vi "E709_Sample_Application_2a.vi"(11 "error in":errorcluster) -> (15 "error out":errorcluster)   [LabVIEW 2014, in "PiFOC.lvlib"]
doc: "This VI demonstrates how to statically define an E-709 configuration with two E 709 controllers. \nIn this example, the first E-709 is connected through COM port 1 with baudrate 115200 and the second through USB with an unknown serial number (Search? = TRUE). The VI runs \"E709_Configuration_Setup.vi\" for both controllers with these pre-defined settings and reads the position of the axes. The diagram shows how to combine the driver VIs for these tasks.\n\nWarning: This VI has Interface settings for each controller that probably do not match your current configuration. Please modify the \"Interface\", \"RS232 settings\" or \"USB settings\" in the diagram before running the VI."
uses:
  PiFOC.lvlib
panel:
  in  "stop":bool
  out "Position system 2":dbl[](array[numeric]) format="%.6f"
  out "Identification E-709 controller 2":string
  out "Conn. Axis system 2":string[](array[string])
  out "Running":bool caption="Axes are referencing"
  out "Position system 1":dbl[](array[numeric]) format="%.6f"
  out "Conn. Axis system 1":string[](array[string])
  out "Identification E-709 controller 1":string
  # "Simple E-709 sample program"
  # "This VI demonstrates how to statically define an E-709 configuration with two E-709 controllers. In this example, the first E-709 is connected through COM\nport 1 with baudrate 57600 and the second through USB. The VI runs E709_Configuration_Setup.vi for both controllers with these pre-defined settings \nand reads the position of the axes. The diagram shows how to combine the driver VIs for these tasks. \n\nWarning: This VI has Interface settings for each controller that probably do not match your current configuration. Please modify the \n                 \"Interface\", \"RS232 settings\" or USB settings\" in the diagram before running the VI."
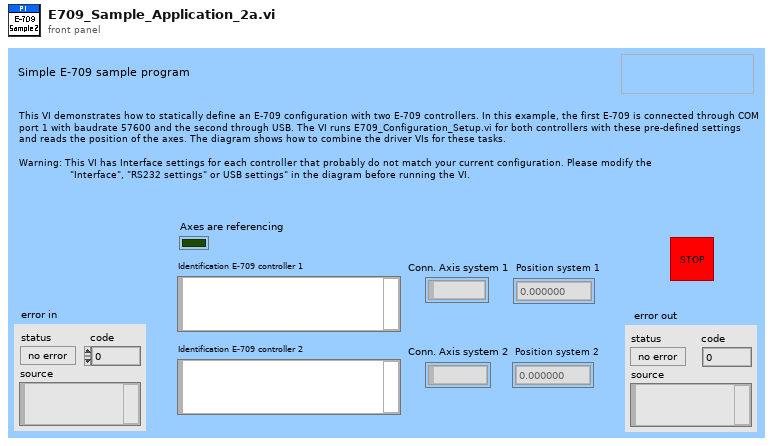
[diagram p1: front panel]
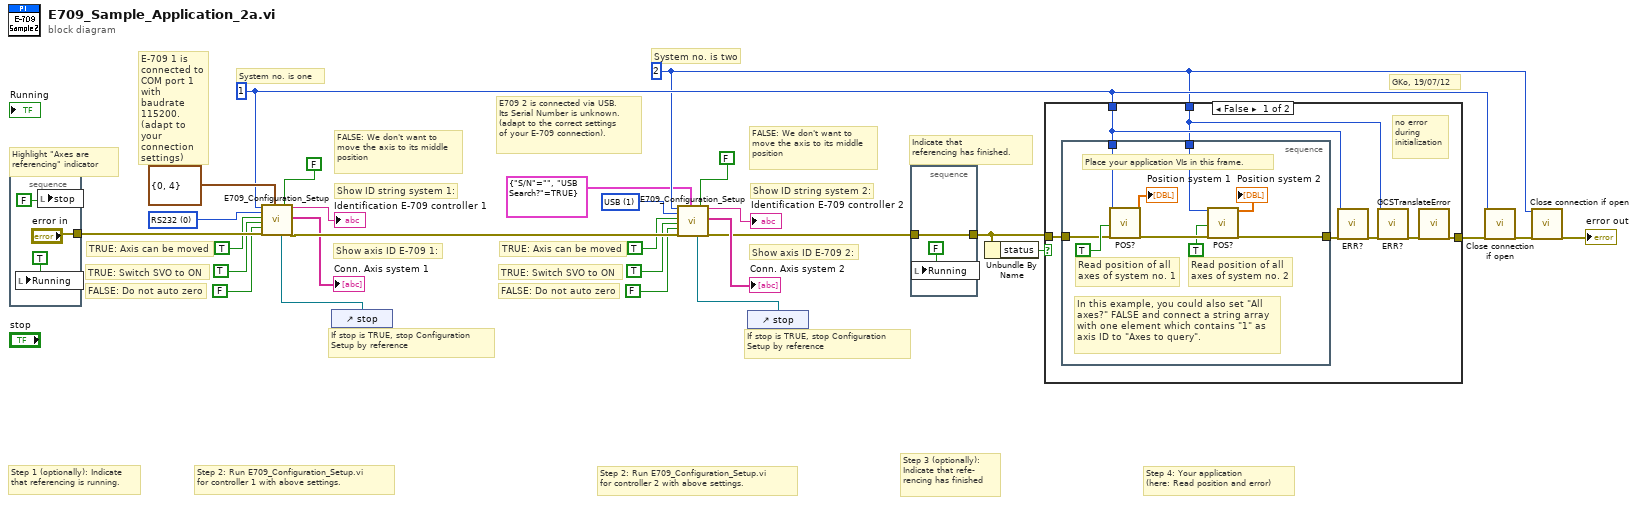
[diagram p0: block diagram]
diagram:
  w1 = u16 1 items=["RS232", "USB", "RS232 DaisyChain"] ("Interface")
  w2 = u16 0 items=["RS232", "USB", "RS232 DaisyChain"] ("Interface")
  w4 = 2 ("System no.")
  w5 = 1 ("System no.")
  # "FALSE: Do not auto zero"
  # "TRUE: Switch SVO to ON"
  # "TRUE: Axis can be moved"
  # "FALSE: Do not auto zero"
  # "TRUE: Switch SVO to ON"
  # "FALSE: We don't want to\nmove the axis to its middle\nposition"
  # "Step 4: Your application\n(here: Read position and error)"
  # "E709 2 is connected via USB.\nIts Serial Number is unknown.\n(adapt to the correct settings\nof your E-709 connection)."
  # "E-709 1 is\nconnected to\nCOM port 1\nwith baudrate\n115200.\n(adapt to your\nconnection\nsettings)"
  # "If stop is TRUE, stop Configuration\nSetup by reference"
  # "If stop is TRUE, stop Configuration\nSetup by reference"
  # "Step 2: Run E709_Configuration_Setup.vi\nfor controller 2 with above settings."
  # "Show axis ID E-709 2:"
  # "Show ID string system 2:"
  # "System no. is two"
  # "GKo, 19/07/12"
  # "Step 3 (optionally): \nIndicate that refe-\nrencing has finished"
  # "Step 2: Run E709_Configuration_Setup.vi\nfor controller 1 with above settings."
  # "Step 1 (optionally): Indicate\nthat referencing is running."
  # "Indicate that\nreferencing has finished."
  # "Highlight \"Axes are\nreferencing\" indicator"
  # "Show axis ID E-709 1:"
  # "Show ID string system 1:"
  # "FALSE: We don't want to\nmove the axis to its middle\nposition"
  # "TRUE: Axis can be moved"
  # "System no. is one"
  n1 = stacked-sequence {
    tunnel: ["error in"] -> w27
    frame #0 {
      n2 = local write "Running"(TRUE ("Running")) -> ()
      n3 = local write "stop"(FALSE ("stop")) -> ()
    }
  }
  n4 = control-ref of="stop"() -> (w22:refnum<vi>)
  n5 = call "E709_Configuration_Setup.vi"("System no."=w5, "Interface"=w2, "Connected?"=TRUE ("All axes?"), "Change servo status to ON?"=TRUE ("Use dialog to define\nconnected stages?"), "Perform autozero?"=FALSE ("Use dialog to define\nconnected stages?"), "error in"=w27, "RS232 settings"=cluster{"Portnumber":i32, "Baudrate":u16} {"Portnumber"=0, "Baudrate"=4}, "Move to middle?"=FALSE ("Use dialog to define\nconnected stages?"), "Stop refnum"=w22) -> ("Identification"=→"Identification E-709 controller 1":string, "Conn. \nAxis"=→"Conn. Axis system 1":string[], "error out"=w24:errorcluster)  [unwired: 5 in, 3 out]
  n6 = control-ref of="stop"() -> (w21:refnum<vi>)
  n7 = call "E709_Configuration_Setup.vi"("System no."=w4, "Interface"=w1, "Connected?"=TRUE ("All axes?"), "Change servo status to ON?"=TRUE ("Use dialog to define\nconnected stages?"), "Perform autozero?"=FALSE ("Use dialog to define\nconnected stages?"), "error in"=w24, "USB settings"=cluster{"S/N":string, "USB Search?":bool} {"S/N"="", "USB Search?"=TRUE}, "Move to middle?"=FALSE ("Use dialog to define\nconnected stages?"), "Stop refnum"=w21) -> ("Identification"=→"Identification E-709 controller 2":string, "Conn. \nAxis"=→"Conn. Axis system 2":string[], "error out"=w23:errorcluster)  [unwired: 5 in, 3 out]
  n8 = stacked-sequence {
    tunnel: w23 -> [w33]
    tunnel: [w33] -> w18
    frame #0 {
      n9 = local write "Running"(FALSE ("Running")) -> ()
    }
  }
  n10 = Unbundle By Name(w18) -> ("status"=w19:bool)
  n11 = case shown="False" w19 {
    tunnel: w5 -> [w35 _]
    tunnel: w18 -> [w40 w50]
    tunnel: [w38 w50] -> w6
    tunnel: w4 -> [w34 _]
    frame False {
      # "no error\nduring\ninitialization"
      n12 = stacked-sequence {
        tunnel: w35 -> [w49]
        tunnel: [w43] -> w39
        tunnel: w40 -> [w47]
        tunnel: w34 -> [w41]
        frame #0 {
          # "Read position of all\naxes of system no. 2"
          # "Read position of all \naxes of system no. 1"
          # "Place your application VIs in this frame."
          # "In this example, you could also set \"All \naxes?\" FALSE and connect a string array \nwith one element which contains \"1\" as \naxis ID to \"Axes to query\"."
          n13 = call "POS?.vi"("System no."=w49, "All axes?"=TRUE, "error in"=w47) -> ("Position"=→"Position system 1":dbl[], "error out"=w44:errorcluster)  [unwired: 2 in, 13 out]
          n14 = call "POS?.vi"("System no."=w41, "All axes?"=TRUE, "error in"=w44) -> ("Position"=→"Position system 2":dbl[], "error out"=w43:errorcluster)  [unwired: 2 in, 13 out]
        }
      }
      n15 = call "ERR?.vi"("System no."=w35, "error in"=w39) -> ("error out"=w37:errorcluster)  [unwired: 17 out]
      n16 = call "ERR?.vi"("System no."=w34, "error in"=w37) -> ("error out"=w36:errorcluster)  [unwired: 17 out]
      n17 = call "GCSTranslateError.vi"("error in"=w36) -> ("error out"=w38:errorcluster)  [unwired: 18 out]
    }
    frame True {
      # "error during initialization!"
    }
  }
  n18 = call "Close connection if open.vi"("System no."=w5, "error in"=w6) -> ("error out"=w8:errorcluster)  [unwired: 1 in, 16 out]
  n19 = call "Close connection if open.vi"("System no."=w4, "error in"=w8) -> ("error out"=→"error out":errorcluster)  [unwired: 1 in, 16 out]
